vi "Load.vi"(7 "Mutable (F)":bool, 8 "error in (no error)":errorcluster, 11 "Config Storage in":refnum<class "Config Storage.lvclass">) -> (0 "error out":errorcluster, 2 "Config":refnum<class "Config Manager.lvclass">, 3 "Config Storage out":refnum<class "Config Storage.lvclass">)   [LabVIEW 2023, in "CDM-Config.lvlib" / "Config Storage.lvclass"]
doc: "Loads the config as saved from the storage implementation. If saved with filters (perhaps as an overlay) then only the filtered portion will be loaded which will be a specific subtree that was saved and/or specific meta fields. For reloading filtered config overlays, <b>Load Overlays</b> should generally be used which will automatically load into an existing base config. Loading overlays explicitly allows modifying the config before its merged in which may be easier on a subset of the full config."
uses:
  Config Storage.lvclass
  Config Manager/Config Manager.lvclass
  Config Storage.lvclass/Config Storage.ctl
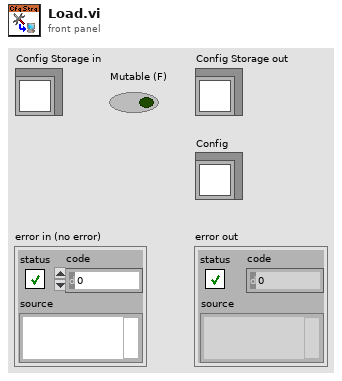
[diagram p1: front panel]
types:
  T1 = typedef "CDM-Config.lvlib/Config Element.ctl" = cluster{"Hierarchy":string[], "Value":variant, "Meta Data":T2[], "Value Type":T3, "Child Order":i32}
  T2 = typedef "CDM-Config.lvlib/Meta Data.ctl" = cluster{"Name":string, "Value":string}
  T3 = typedef "CDM-Config.lvlib/Value Type.ctl" = enum16{"String", "Number", "Bool", "Object", "Array"}
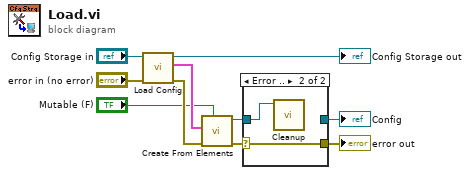
[diagram p0: block diagram]
diagram:
  n1 = call-dynamic "Load Config.vi"("error in (no error)"="error in (no error)", "Config Storage in"="Config Storage in") -> ("error out"=w6:errorcluster, "Elements"=w7:T1[], "Config Storage out"=→"Config Storage out":refnum<class "Config Storage.lvclass">)  [unwired: 7 in]
  n2 = call "Create From Elements.vi"("Mutable (F)"="Mutable (F)", "error in (no error)"=w6, "Elements"=w7) -> ("error out"=w5:errorcluster, "Config Manager out"=w3:refnum<class "Config Manager.lvclass">)  [unwired: 7 in]
  n3 = case shown="Error .." w5 {
    selector: w5 -> [w11 w13]
    tunnel: [w11 w13] -> w4
    tunnel: w3 -> [w12 w14]
    tunnel: [w12 _] -> w2
    frame No Error {
    }
    frame Error {
      n4 = call "Cleanup.vi"("Config Manager in"=w14) -> ()  [unwired: 10 in, 1 out]
    }
  }
  "error out" <- w4
  "Config" <- w2
